vi "Monitor console output and wait for one of many keywords.vi"(5 "Wait msecs after cmd ends (500ms)":u32=500, 6 "VISA resource name":refnum<visa-resource-name>, 7 "Timeout (1000 mSecs)":u32=1000, 8 "error in (no error)":errorcluster, 9 "Wait for keywords":string[](array[string]), 11 "Wait after send":u32=750) -> (0 "error out":errorcluster, 1 "Response":string, 2 "Keyword found index":i32, 3 "Found key?":bool, 4 "VISA Refnum out":refnum<visa-resource-name>)   [LabVIEW 2024]
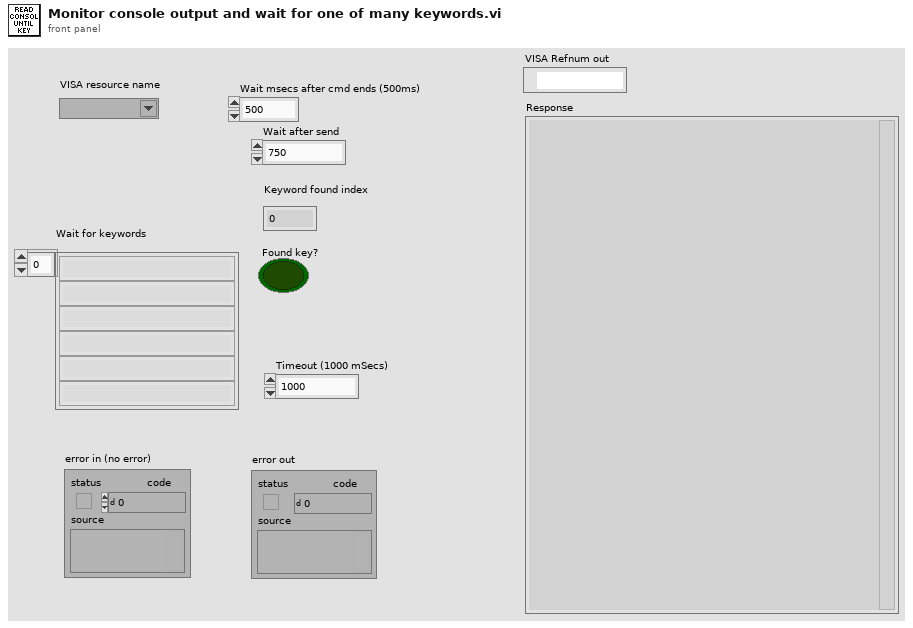
[diagram p1: front panel]
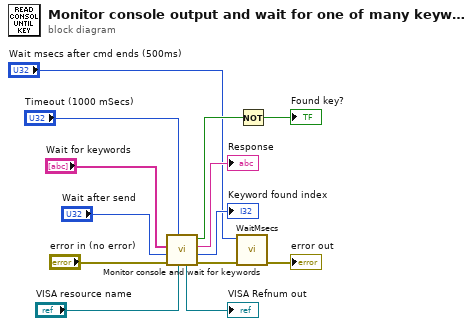
[diagram p0: block diagram]
diagram:
  n1 = call "Monitor console and wait for keywords.vi"("VISA resource name"="VISA resource name", "Timeout (mSecs)"="Timeout (1000 mSecs)", "error in (no error)"="error in (no error)", "Wait after"="Wait after send", "Wait for keywords"="Wait for keywords") -> ("error out"=w5:errorcluster, "Keyword found index"=→"Keyword found index":i32, "Response"=→"Response":string, "timeout"=w8:bool, "VISA Refnum out"=→"VISA Refnum out":refnum<visa-resource-name>)  [unwired: 2 in]
  n2 = call "WaitMsecs.vi"("error in (no error)"=w5, "Wait Msecs"="Wait msecs after cmd ends (500ms)") -> ("error out"=→"error out":errorcluster)  [unwired: 9 in]
  n3 = Not(x=w8) -> (.not. x?=→"Found key?":bool)
